vi "Test Initialize Subpanels.vi"(8 "error in":errorcluster) -> (0 "error out":errorcluster)   [LabVIEW 2020]
uses:
  Maui Manager/Maui Manager.lvclass
  Maui Manager/Maui Manager.lvclass/Maui Manager.ctl
  <vilib>/addons/_JKI Toolkits/Caraya/classes/Assert/Assert Equal Value_Variant.vi
  <vilib>/addons/_JKI Toolkits/Caraya/classes/Assert/Assert.lvclass
  <vilib>/addons/_JKI Toolkits/Caraya/classes/Test/Test.lvclass
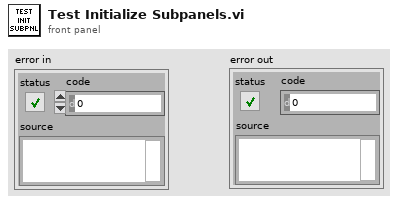
[diagram p1: front panel]
types:
  T1 = cluster{"Control":refnum<vi>, "Subpanel":refnum<vi>, "Active":i32, "Ctrl Class":string}[]
  T2 = cluster{"Control":refnum<vi>, "Subpanel":refnum<vi>, "Active":i32, "Ctrl Class":string}
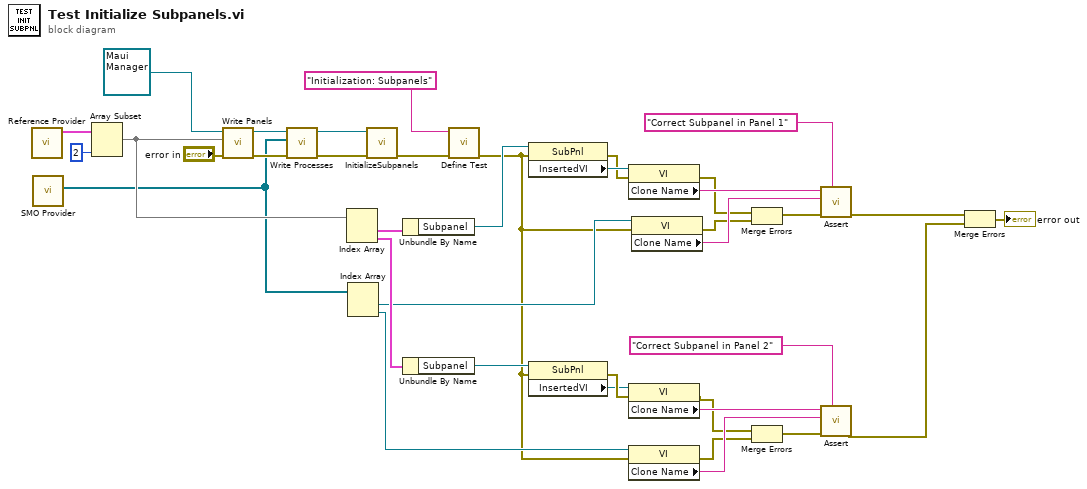
[diagram p0: block diagram]
diagram:
  n1 = call "Reference Provider.vi"() -> ("References"=w37:T1)  [unwired: 11 in]
  n2 = call "SMO Provider.vi"() -> ("Refs"=w24:refnum<vi>[])  [unwired: 10 in, 1 out]
  n3 = Array Subset(array=w37, length=2) -> (w32:T1)  [unwired: 1 in]
  n4 = call "Write Panels.vi"("error in (no error)"="error in", "Panels"=w32, "Maui Manager in"=refnum<class "Maui Manager.lvclass"> refnum ("Maui Manager.lvclass")) -> ("error out"=w34:errorcluster, "Maui Manager out"=w35:refnum<class "Maui Manager.lvclass">)  [unwired: 7 in]
  n5 = call "Write Processes.vi"("error in (no error)"=w34, "Processes"=w24, "Maui Manager in"=w35) -> ("error out"=w30:errorcluster, "Maui Manager out"=w31:refnum<class "Maui Manager.lvclass">)  [unwired: 7 in]
  n6 = Index Array(array=w32) -> (element #1=w28:T2, element #2=w23:T2)  [unwired: 2 in]
  n7 = Index Array(array=w24) -> (element #1=w19:refnum<vi>, element #2=w18:refnum<vi>)  [unwired: 2 in]
  n8 = call "InitializeSubpanels.vi"("error in (no error)"=w30, "Maui Manager in"=w31) -> ("error out"=w29:errorcluster)  [unwired: 8 in, 1 out]
  n9 = Unbundle By Name(w28) -> ("Subpanel"=w27:refnum<vi>)
  n10 = Unbundle By Name(w23) -> ("Subpanel"=w20:refnum<vi>)
  n11 = call <vilib>:"Define Test.vi"("error in (no error)"=w29, "Label (VI Title)"="Initialization: Subpanels") -> ("error out"=w10:errorcluster)  [unwired: 9 in]
  n12 = property class="SubPnl"(reference=w27, error in=w10) -> (error out=w25:errorcluster, "InsertedVI"=w26:refnum<vi>)  [unwired: 1 out]
  n13 = property class="SubPnl"(reference=w20, error in=w10) -> (error out=w22:errorcluster, "InsertedVI"=w21:refnum<vi>)  [unwired: 1 out]
  n14 = property class="VI"(reference=w26, error in=w25) -> (error out=w8:errorcluster, "Clone Name"=w17:string)  [unwired: 1 out]
  n15 = property class="VI"(reference=w21, error in=w22) -> (error out=w5:errorcluster, "Clone Name"=w14:string)  [unwired: 1 out]
  n16 = property class="VI"(reference=w18, error in=w10) -> (error out=w4:errorcluster, "Clone Name"=w13:string)  [unwired: 1 out]
  n17 = property class="VI"(reference=w19, error in=w10) -> (error out=w7:errorcluster, "Clone Name"=w16:string)  [unwired: 1 out]
  n18 = Merge Errors(w8, w7) -> (w9:errorcluster)
  n19 = Merge Errors(w5, w4) -> (w6:errorcluster)
  n20 = call-poly <vilib>:"Assert.vi"("Label"="Correct Subpanel in Panel 1", "error in (no error)"=w9, "Y"=w16, "X"=w17) -> ("error out"=w3:errorcluster)  [unwired: 7 in]
  n21 = call-poly <vilib>:"Assert.vi"("Label"="Correct Subpanel in Panel 2", "error in (no error)"=w6, "Y"=w13, "X"=w14) -> ("error out"=w2:errorcluster)  [unwired: 7 in]
  n22 = Merge Errors(w3, w2) -> (→"error out":errorcluster)
